vi "Parsing.vi"(3 "Cluster":T1={"Prefix"="ni.var.psp://", "IP"="", "Librery name"="Shared Variable/", "Variable name"=""}) -> (0 "String":string)   [LabVIEW 2021]
uses:
  Variable custer.ctl
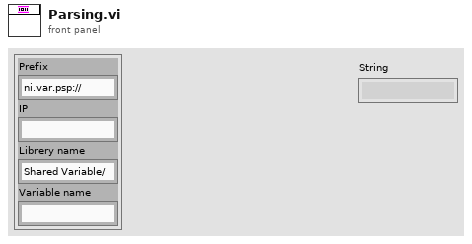
[diagram p1: front panel]
types:
  T1 = typedef "Variable custer.ctl" = cluster{"Prefix":string, "IP":string, "Librery name":string, "Variable name":string}
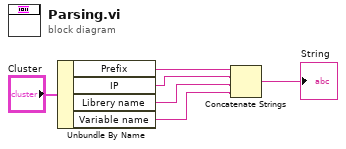
[diagram p0: block diagram]
diagram:
  n1 = Unbundle By Name("Cluster") -> ("Prefix"=w5:string, "IP"=w4:string, "Librery name"=w3:string, "Variable name"=w2:string)
  n2 = Concatenate Strings(w5, w4, w3, w2) -> (→"String":string)
